vi "全局 工程师.vi"() -> ()   [LabVIEW 2011]
panel:
  out "工程师":bool
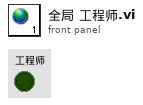
[diagram p1: front panel]
diagram:
